vi "Add to Project.vi"(7 "AppInst":refnum<vi>, 8 "error in (no error)":errorcluster, 9 "Folder":string="MESSAGES FOR THIS ACTOR", 10 "Class Path":path, 11 "Actor":refnum<vi>) -> (0 "error out":errorcluster)   [LabVIEW 2020, in "Message Maker.lvlib"]
uses:
  Message Maker.lvlib
  <vilib>/Utility/EditLVLibs/Edit LVLibs.lvlib
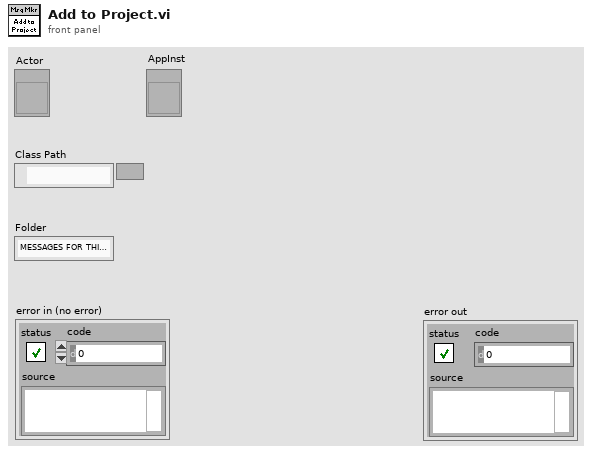
[diagram p1: front panel]
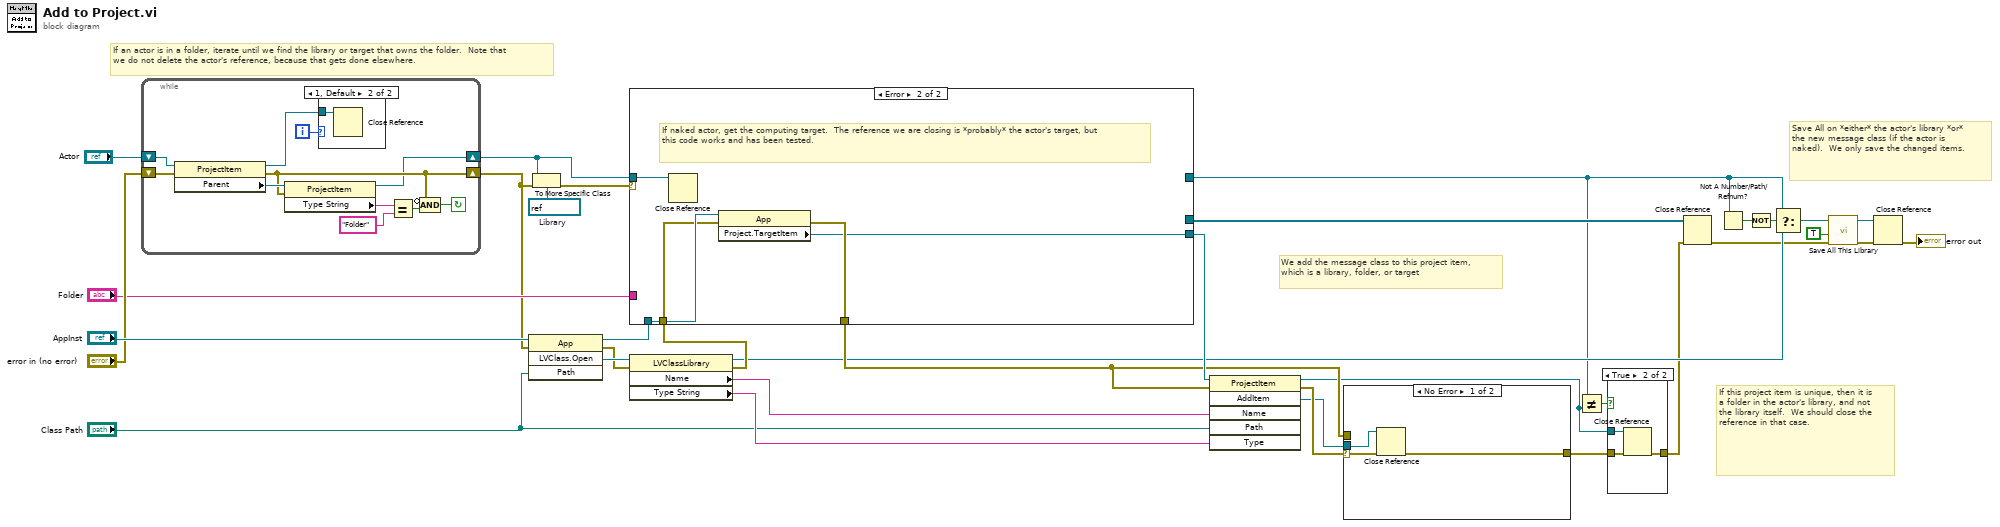
[diagram p0: block diagram]
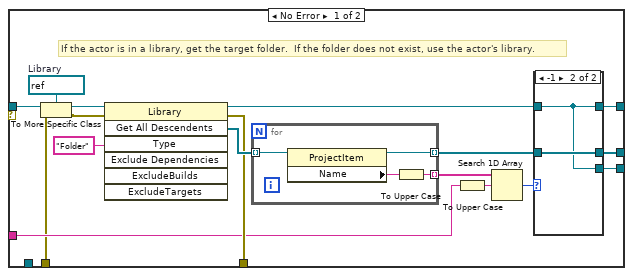
[diagram p4: hidden frame]
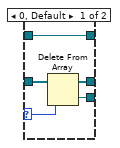
[diagram p5: hidden frame]
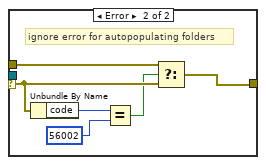
[diagram p6: hidden frame]
diagram:
  w24 = refnum<vi> refnum  # Library
  # "If an actor is in a folder, iterate until we find the library or target that owns the folder.  Note that we do not delete the actor's reference, because that gets done elsewhere."
  # "If this project item is unique, then it is a folder in the actor's library, and not the library itself.  We should close the reference in that case."
  # "Save All on *either* the actor's library *or* the new message class (if the actor is naked).  We only save the changed items."
  # "We add the message class to this project item, which is a library, folder, or target"
  n1 = while {
    shift-right: [w39] -> w5
    shift-left: "error in (no error)" -> [w44]
    shift-right: [w35] -> w4
    shift-left: "Actor" -> [w45]
    i -> [w36]
    stop <- w38 continue-if-true
    n2 = property class="ProjectItem"(reference=w45, error in=w44) -> (reference out=w37:refnum<vi>, error out=w39:errorcluster, "Parent"=w43:refnum<vi>)
    n3 = property class="ProjectItem"(reference=w43, error in=w39) -> (reference out=w35:refnum<vi>, "Type String"=w42:string)  [unwired: 1 out]
    n4 = case shown="1, Default" w36 {
      tunnel: w37 -> [_ w46]
      frame 0 {
      }
      frame 1, Default {
        n5 = Close Reference(reference=w46) -> ()  [unwired: 1 in, 1 out]
      }
    }
    n6 = Equal?(x=w42, y="Folder") -> (x = y?=w40:bool)
    n7 = Compound Arithmetic op=AND(invert w39, w40) -> (w38:bool)
  }
  n8 = invoke class="App" method="LVClass.Open"(reference="AppInst", error in=w5, "Path"="Class Path") -> (reference out=w21:refnum<vi>, error out=w33:errorcluster, "LVClass.Open"=w34:refnum<vi>)  [unwired: 1 in, 1 out]
  n9 = To More Specific Class(target class=w24, reference=w4, error in=w5) -> (error out=w23:errorcluster)  [unwired: 1 out]
  n10 = property class="LVClassLibrary"(reference=w34, error in=w33) -> (reference out=w11:refnum<vi>, error out=w22:errorcluster, "Name"=w32:string, "Type String"=w31:string)
  n11 = case shown="Error" w23 {
    tunnel: [w58 _] -> w27
    tunnel: [w57 w76] -> w25
    tunnel: w4 -> [w51 w75]
    tunnel: w22 -> [w49 w78]
    tunnel: [w56 w77] -> w17
    tunnel: w21 -> [_ w79]
    tunnel: "Folder" -> [w55 _]
    tunnel: [w53 _] -> w1
    frame No Error {
      w48 = refnum<vi> refnum  # Library
      # "If the actor is in a library, get the target folder.  If the folder does not exist, use the actor's library."
      n12 = To More Specific Class(target class=w48, reference=w51, error in=w49) -> (specific class reference=w50:refnum<vi>, error out=w47:errorcluster)
      n13 = invoke class="Library" method="Get All Descendents"(reference=w50, error in=w47, "Type"="Folder") -> (reference out=w54:refnum<vi>, error out=w56:errorcluster, "All Descendents"=w62:refnum<vi>[])  [unwired: 4 in, 4 out]
      n14 = for {
        tunnel: [w71] -> w61 mode=indexing
        tunnel: w62 -> [w73] mode=indexing
        tunnel: [w72] -> w59 mode=indexing
        n15 = property class="ProjectItem"(reference=w73) -> (reference out=w72:refnum<vi>, "Name"=w74:string)  [unwired: 1 in, 1 out]
        n16 = To Upper Case(1:w74) -> (0:w71:string)
      }
      n17 = To Upper Case(1:w55) -> (0:w52:string)
      n18 = Search 1D Array(1D array=w61, element=w52) -> (index of element=w60:i32)  [unwired: 1 in]
      n19 = case shown="-1" w60 {
        selector: w60 -> [w68 _]
        tunnel: w59 -> [w66 w70]
        tunnel: w54 -> [w64 w69]
        tunnel: [w67 w69] -> w57
        tunnel: [w65 w70] -> w58
        tunnel: [w64 w69] -> w53
        frame 0, Default {
          n20 = Delete From Array(array=w66, index=w68) -> (deleted portion=w67:refnum<vi>, array with subset deleted=w65:refnum<vi>[])  [unwired: 1 in]
        }
        frame -1 {
        }
      }
    }
    frame Error {
      # "If naked actor, get the computing target.  The reference we are closing is *probably* the actor's target, but this code works and has been tested."
      n21 = Close Reference(reference=w75) -> ()  [unwired: 1 in, 1 out]
      n22 = property class="App"(reference=w79, error in=w78) -> (error out=w77:errorcluster, "Project.TargetItem"=w76:refnum<vi>)  [unwired: 1 out]
    }
  }
  n23 = invoke class="ProjectItem" method="AddItem"(reference=w25, error in=w17, "Name"=w32, "Path"="Class Path", "Type"=w31) -> (reference out=w2:refnum<vi>, error out=w29:errorcluster, "AddItem"=w18:refnum<vi>)  [unwired: 1 in, 3 out]
  n24 = case shown="No Error" w29 {
    selector: w29 -> [w82 w85]
    tunnel: w17 -> [_ w86]
    tunnel: [w80 w84] -> w8
    tunnel: w18 -> [w81 _]
    frame No Error {
      n25 = Close Reference(reference=w81, error in (no error)=w82) -> (error out=w80:errorcluster)
    }
    frame Error {
      # "ignore error for autopopulating folders"
      n26 = Unbundle By Name(w85) -> ("code"=w88:i32)
      n27 = Equal?(x=w88, y=56002) -> (x = y?=w83:bool)
      n28 = Select(t=w86, s=w83, f=w85) -> (s? t:f=w84:errorcluster)
    }
  }
  n29 = Not Equal?(x=w1, y=w2) -> (x != y?=w3:bool)
  n30 = case shown="True" w3 {
    tunnel: [w89 w92] -> w9
    tunnel: w8 -> [w89 w91]
    tunnel: w2 -> [_ w90]
    frame False {
    }
    frame True {
      n31 = Close Reference(reference=w90, error in (no error)=w91) -> (error out=w92:errorcluster)
    }
  }
  n32 = Close Reference(reference=w27, error in (no error)=w9) -> (error out=w7:errorcluster)
  n33 = Not A Number/Path/Refnum?(number/path/refnum=w1) -> (NaN/Path/Refnum?=w13:bool)
  n34 = Not(x=w13) -> (.not. x?=w12:bool)
  n35 = Select(t=w1, s=w12, f=w11) -> (s? t:f=w10:refnum<vi>)
  n36 = call <vilib>:"Save All This Library.vi"("error in (no error)"=w7, "Save Only Modified VIs and Libraries? (F)"=TRUE ("Save Only Modified VIs? (F)"), "Library in"=w10) -> ("error out"=w15:errorcluster, "Library out"=w14:refnum<vi>)  [unwired: 7 in]
  n37 = Close Reference(reference=w14, error in (no error)=w15) -> (error out=→"error out":errorcluster)
